vi "result.To JSON String.vi"(8 "error in (no error)":errorcluster, 11 "result in":refnum<class "result.lvclass">) -> (0 "error out":errorcluster, 2 "JSON String":string, 3 "result out":refnum<class "result.lvclass">)   [LabVIEW 2016, in "result.lvclass"]
uses:
  result.lvclass
  <vilib>/NI/JSON Support for LabVIEW/JSON Value/JSON Value.lvclass
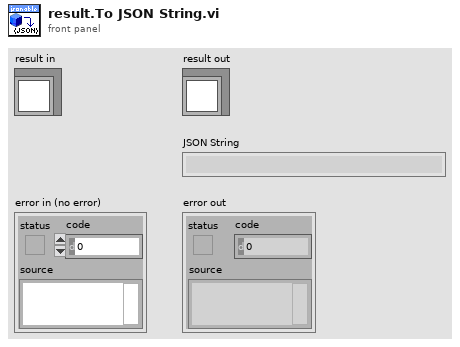
[diagram p1: front panel]
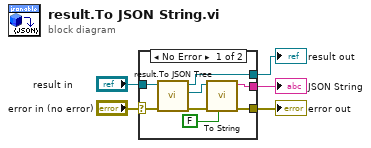
[diagram p0: block diagram]
diagram:
  n1 = case shown="No Error" "error in (no error)" {
    selector: "error in (no error)" -> [w12 w15]
    tunnel: [w8 w15] -> w4
    tunnel: [w11 w14] -> w2
    tunnel: "result in" -> [w13 w14]
    tunnel: [w9 _] -> w1
    frame No Error {
      n2 = call "result.To JSON Tree.vi"("error in (no error)"=w12, "result in"=w13) -> ("error out"=w7:errorcluster, "JSON Value out"=w10:refnum<class "JSON Value.lvclass">, "result out"=w11:refnum<class "result.lvclass">)  [unwired: 7 in]
      n3 = call <vilib>:"To String.vi"("pretty print? (F)"=FALSE ("pretty print? (T)"), "error in (no error)"=w7, "JSON Value in"=w10) -> ("error out"=w8:errorcluster, "String"=w9:string)  [unwired: 7 in]
    }
    frame Error {
    }
  }
  "error out" <- w4
  "result out" <- w2
  "JSON String" <- w1
